vi "Resonance Detector Create sp_dat.vi"(8 "Error In":errorcluster, 10 "Fit results":dbl[][](array[numeric]) format="%#_4p", 11 "File Path Control":path) -> (0 "Error Out":errorcluster)   [LabVIEW 2016]
uses:
  <vilib>/Utility/file.llb/Write Delimited Spreadsheet (DBL).vi
panel:
  out "subarray":dbl[][](array[numeric])
  # "F0         dF     Ampl   Phase   Xbgrd   Ybgrd"
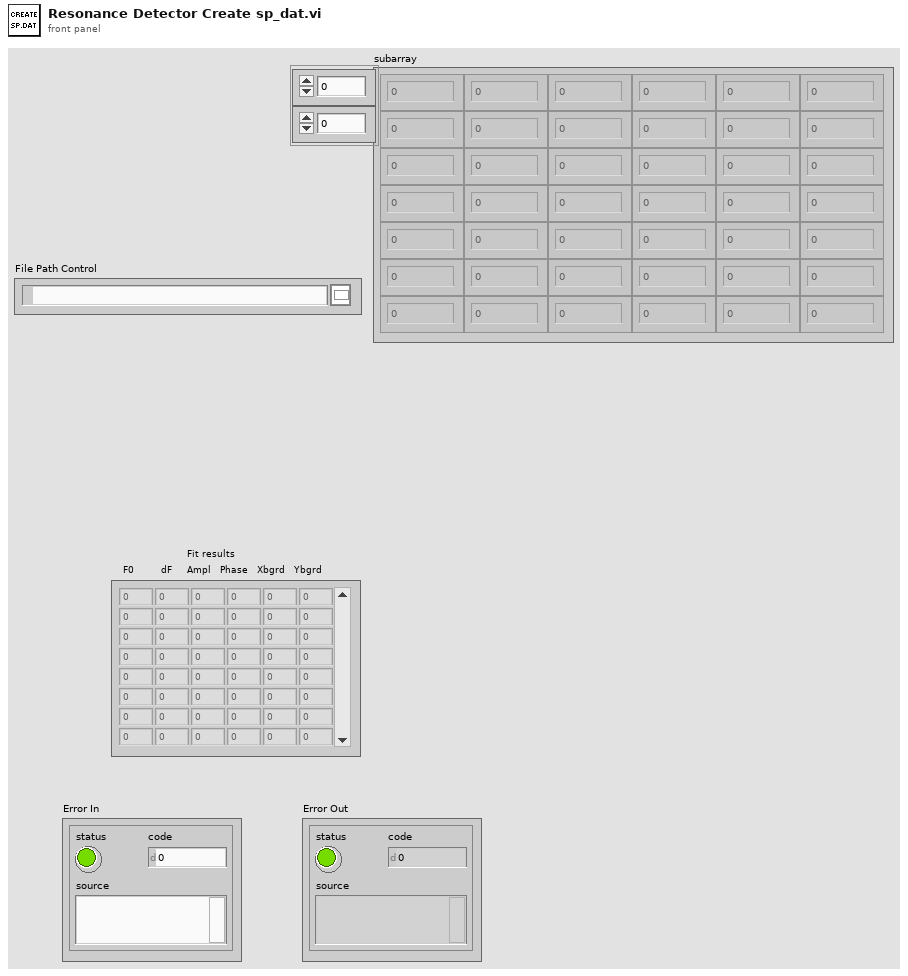
[diagram p1: front panel]
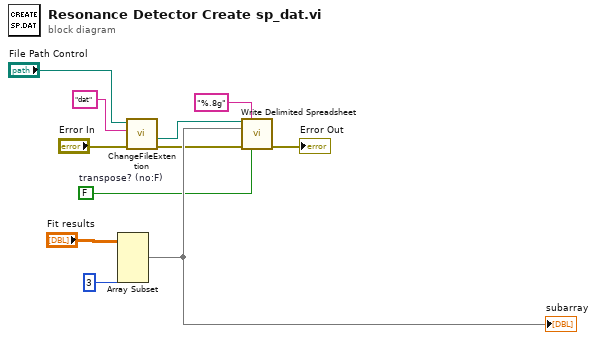
[diagram p0: block diagram]
diagram:
  w3 = FALSE  # transpose? (no:F)
  n1 = Array Subset(array="Fit results", length (col)=3 ("length")) -> (w4:dbl[][])  [unwired: 3 in]
  "subarray" <- w4
  n2 = call "ChangeFileExtention.vi"("Error In"="Error In", "New extension"="dat", "File Path"="File Path Control") -> ("Error Out"=w2:errorcluster, "Path with new extension"=w5:path)  [unwired: 3 in, 4 out]
  n3 = call-poly <vilib>:"Write Delimited Spreadsheet.vi"("file path (dialog if empty)"=w5, "format (%.3f)"="%.8g", "2D data"=w4, "error in (no error)"=w2, "transpose? (no:F)"=w3) -> ("error out"=→"Error Out":errorcluster)  [unwired: 9 in, 1 out]
